vi "XMLRelult_Save_To_File2.vi"(10 "INT DATA":string[][](array[string]), 11 "XML File Path":path caption="XML文件路径") -> (2 "连接的字符串":string, 3 "XML File Path(duplicate)":path caption="XML文件路径（副本）")   [LabVIEW 2018]
uses:
  Subvi/Global.vi
panel:
  out "XML String":string caption="XML字符串"
  in  "INT DATA 3":string[][](array[string])
  in  "INT DATA 2":string[][](array[string])
  out "字符串":string
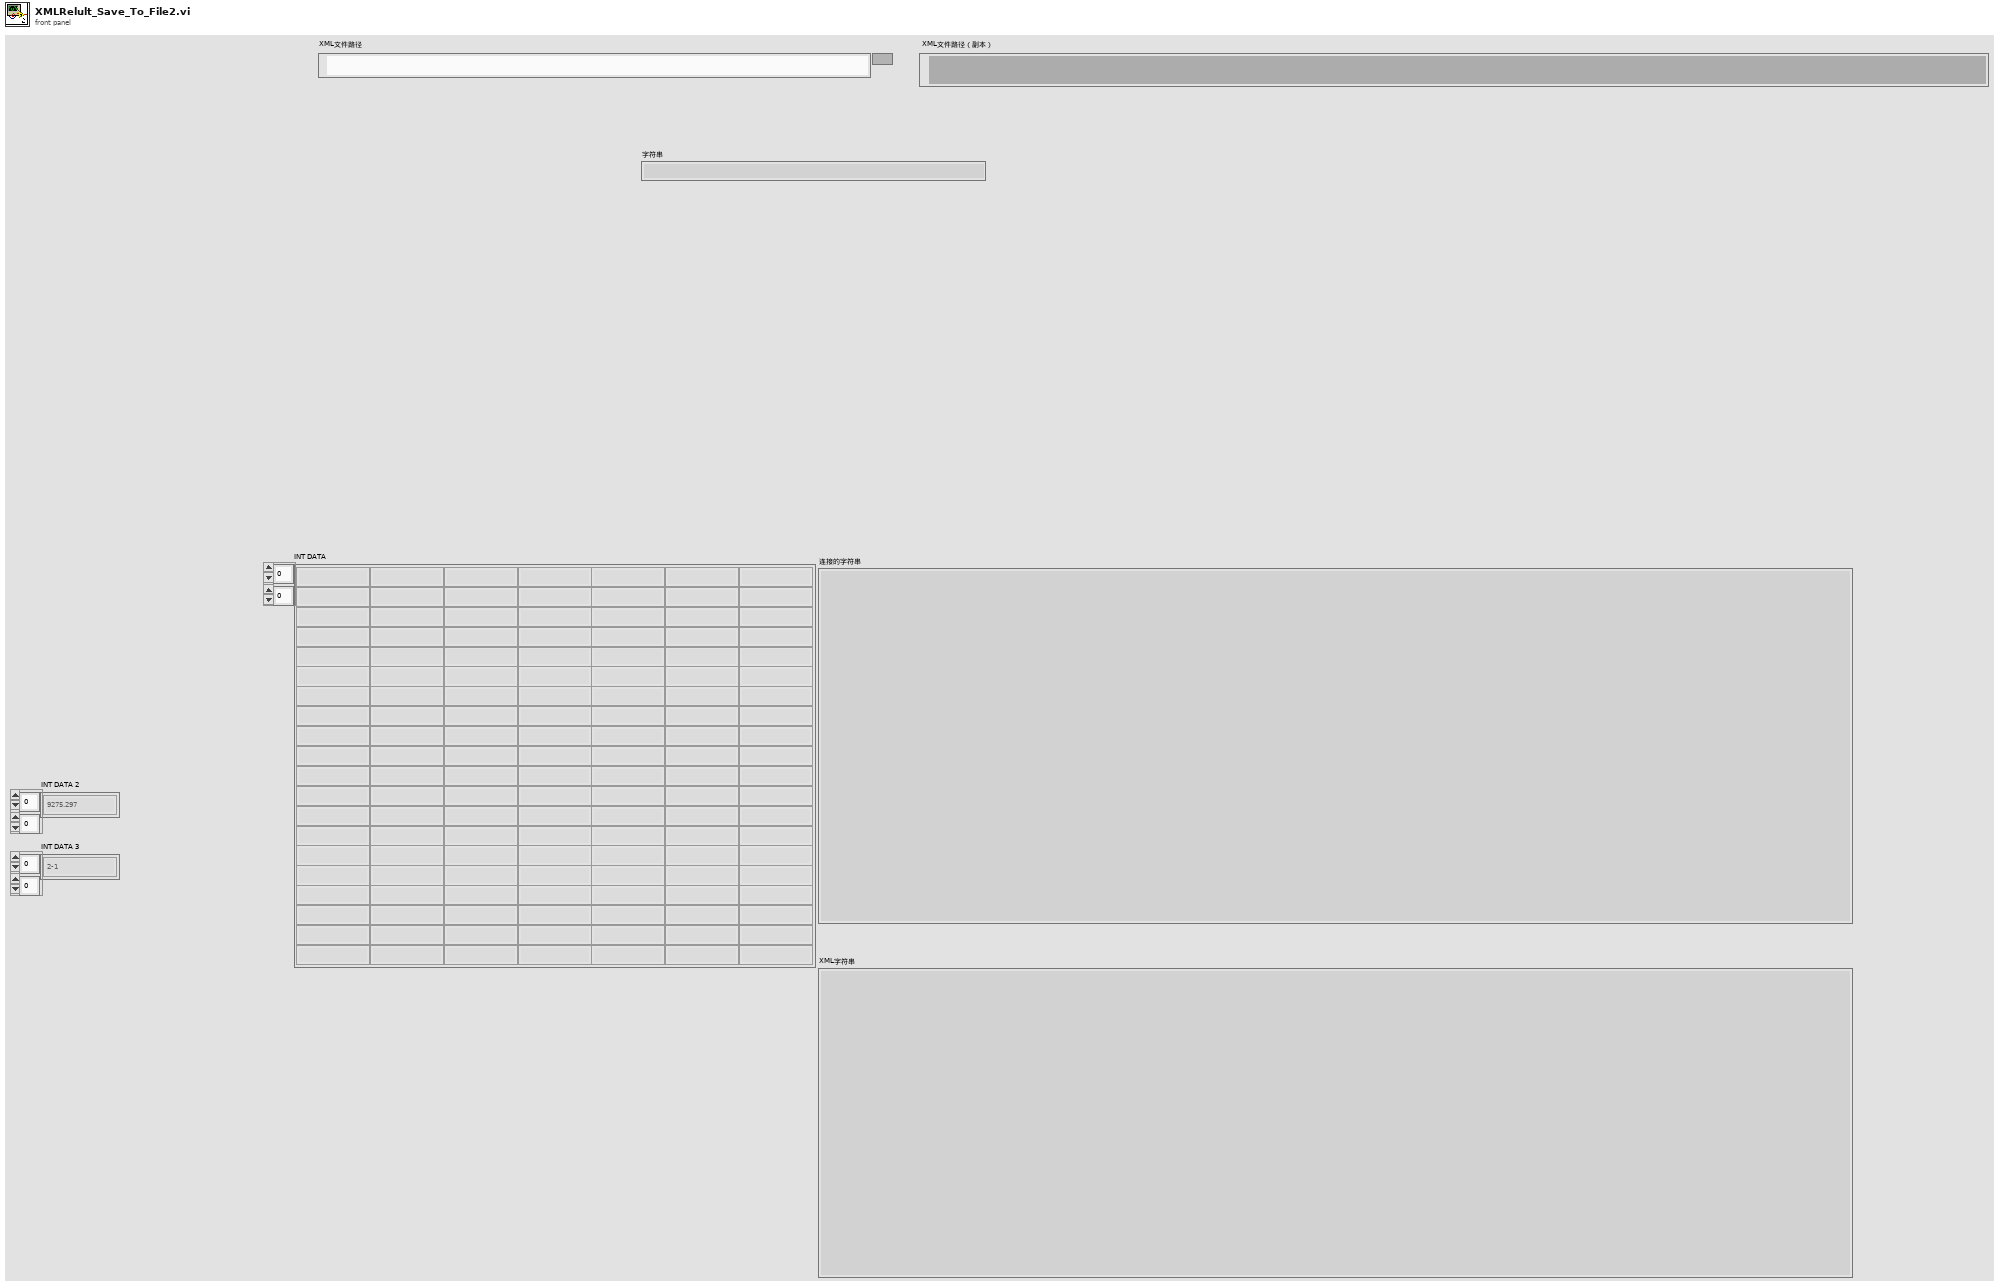
[diagram p1: front panel]
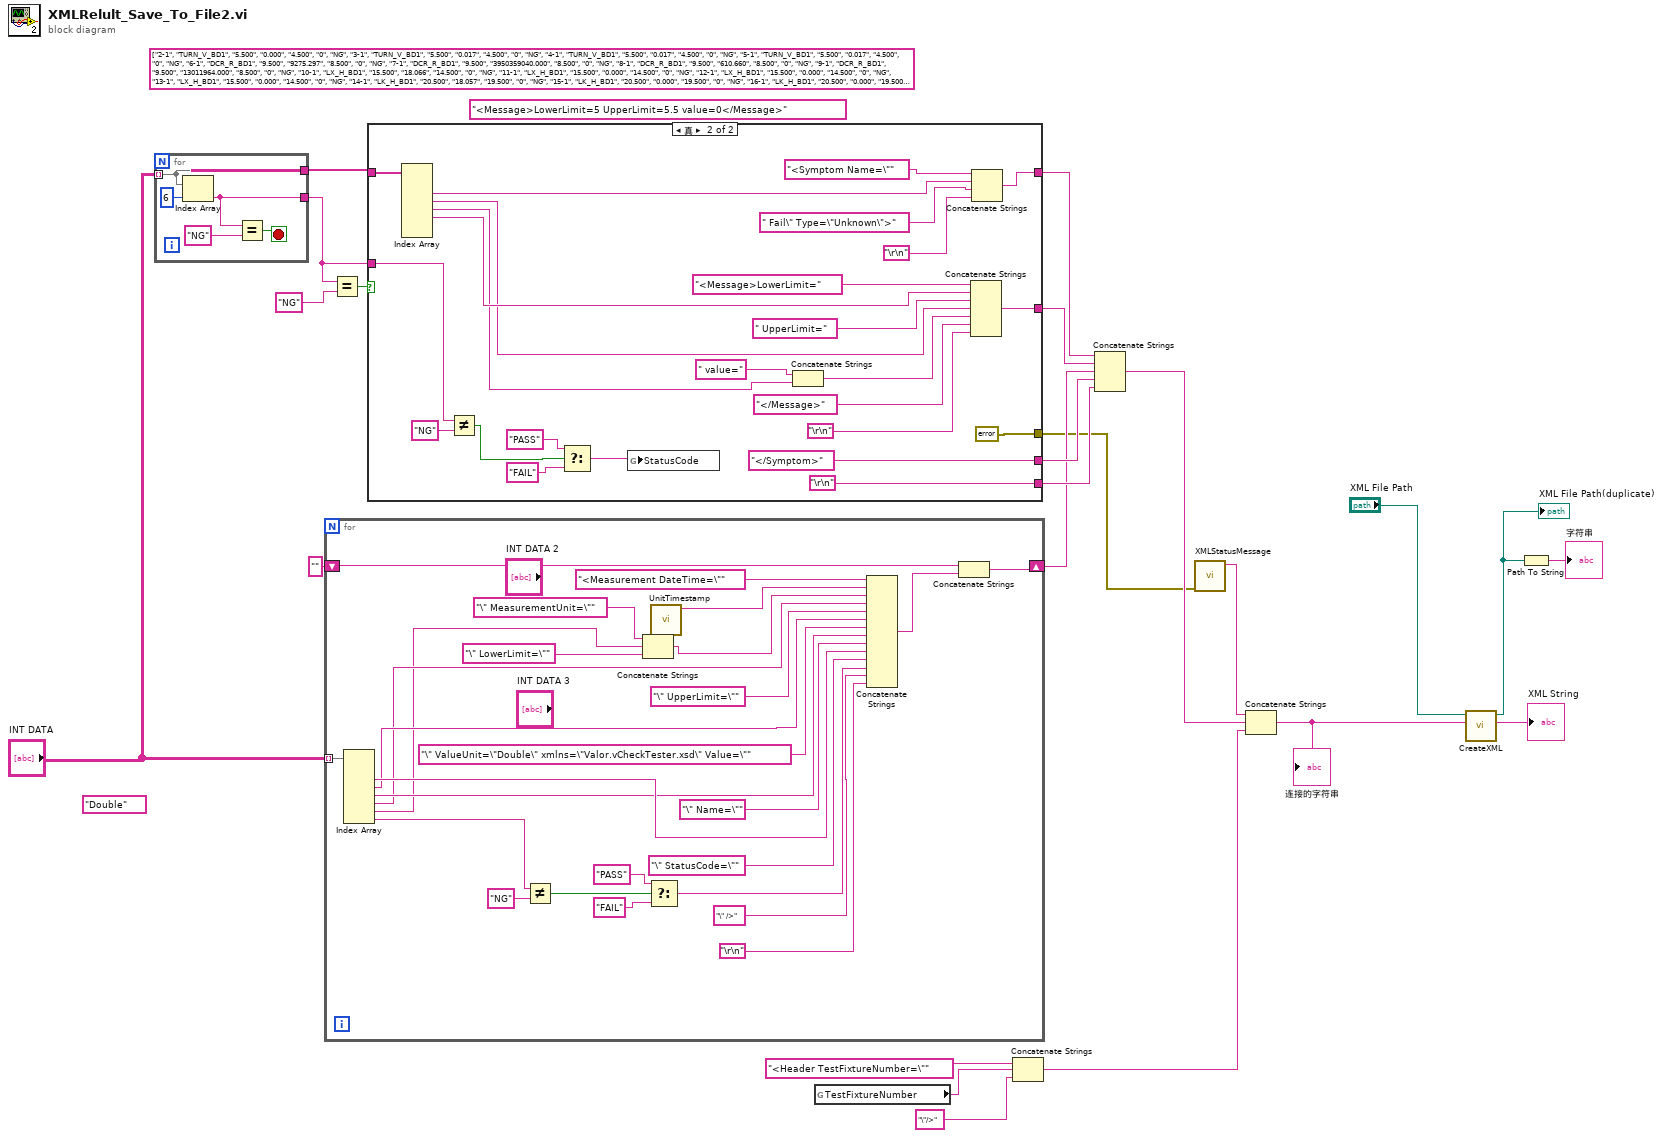
[diagram p0: block diagram]
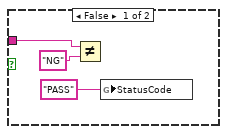
[diagram p2: hidden frame]
diagram:
  (unwired) string[][] [["2-1", "TURN_V_BD1", "5.500", "0.000", "4.500", "0", "NG"], ["3-1", "TURN_V_BD1", "5.500", "0.017", "4.500", "0", "NG"], ["4-1", "TURN_V_BD1", "5.500", "0.017", "4.500", "0", "NG"], ["5-1", "TURN_V_BD1", "5.500", "0.017", "4.500", "0", "NG"], ["6-1", "DCR_R_BD1", "9.500", "9275.297", "8.500", "0", "NG"], ["7-1", "DCR_R_BD1", "9.500", "3950359040.000", "8.500", "0", "NG"], ["8-1", "DCR_R_BD1", "9.500", "610.660", "8.500", "0", "NG"], ["9-1", "DCR_R_BD1", "9.500", "13011964.000", "8.500", "0", "NG"], ["10-1", "LX_H_BD1", "15.500", "18.066", "14.500", "0", "NG"], ["11-1", "LX_H_BD1", "15.500", "0.000", "14.500", "0", "NG"], ["12-1", "LX_H_BD1", "15.500", "0.000", "14.500", "0", "NG"], ["13-1", "LX_H_BD1", "15.500", "0.000", "14.500", "0", "NG"], ["14-1", "LK_H_BD1", "20.500", "18.057", "19.500", "0", "NG"], ["15-1", "LK_H_BD1", "20.500", "0.000", "19.500", "0", "NG"], ["16-1", "LK_H_BD1", "20.500", "0.000", "19.500", "0", "NG"], ["17-1", "LK_H_BD1", "20.500", "0.000", "19.500", "0", "NG"]] ("INT DATA")
  (unwired) "<Message>LowerLimit=5 UpperLimit=5.5 value=0</Message>"
  (unwired) "Double" ("组合框")
  n1 = for {
    tunnel: "INT DATA" -> [w25] mode=indexing
    tunnel: [w25] -> w8
    tunnel: [w24] -> w6
    stop <- w27 stop-if-true
    n2 = Index Array(array=w25, index=6 ("索引")) -> (element=w24:string)
    n3 = Equal?(x=w24, y="NG") -> (x = y?=w27:bool)
  }
  n4 = for {
    tunnel: "INT DATA" -> [w54] mode=indexing
    shift-right: [w40] -> w9
    shift-left: "" ("字符串") -> [w41]
    n5 = Index Array(array=w54) -> (element #2=w33:string, element #3=w31:string, element #4=w32:string, element #5=w30:string, element #6=w29:string, element #7=w35:string)  [unwired: 7 in, 1 out]
    n6 = Not Equal?(x=w35, y="NG") -> (x != y?=w34:bool)
    n7 = Concatenate Strings("\" MeasurementUnit=\"", w29, "\" LowerLimit=\"") -> (w53:string)
    n8 = Select(t="PASS", s=w34, f="FAIL") -> (s? t:f=w37:string)
    n9 = call "UnitTimestamp.vi"() -> ("字符串"=w43:string)  [unwired: 10 in, 1 out]
    n10 = Concatenate Strings("<Measurement DateTime=\"", w43, w53, w30, "\" UpperLimit=\"", w31, "\" ValueUnit=\"Double\" xmlns=\"Valor.vCheckTester.xsd\" Value=\"", w32, "\" Name=\"", w33, "\" StatusCode=\"", w37, "\" />", "\r\n") -> (w50:string)
    n11 = Concatenate Strings(w41, w50) -> (w40:string)
  }
  n12 = Equal?(x=w6, y="NG") -> (x = y?=w7:bool)
  n13 = case shown="真" w7 {
    tunnel: [_ w75] -> w11
    tunnel: [_ w74] -> w12
    tunnel: [_ "</Symptom>"] -> w13
    tunnel: [_ "\r\n"] -> w14
    tunnel: w8 -> [_ w71]
    tunnel: w6 -> [w56 w60]
    tunnel: [_ errorcluster {"status"=FALSE, "code"=0, "source"=""} ("error out")] -> w5
    frame False {
      n14 = Not Equal?(x=w56, y="NG") -> ()  [unwired: 1 out]
      n15 = global write "Global.vi" "StatusCode"("PASS") -> ()
    }
    frame True {
      n16 = Index Array(array=w71) -> (element #2=w70:string, element #3=w68:string, element #4=w66:string, element #5=w69:string)  [unwired: 7 in, 3 out]
      n17 = Not Equal?(x=w60, y="NG") -> (x != y?=w59:bool)
      n18 = Select(t="PASS", s=w59, f="FAIL") -> (s? t:f=w63:string)
      n19 = global write "Global.vi" "StatusCode"(w63) -> ()
      n20 = Concatenate Strings(" value=", w66) -> (w65:string)
      n21 = Concatenate Strings("<Message>LowerLimit=", w69, " UpperLimit=", w68, w65, "</Message>", "\r\n") -> (w75:string)
      n22 = Concatenate Strings("<Symptom Name=\"", w70, " Fail\" Type=\"Unknown\">", "\r\n") -> (w74:string)
    }
  }
  n23 = global read "Global.vi" "TestFixtureNumber"() -> (w21:string)
  n24 = Concatenate Strings("<Header TestFixtureNumber=\"", w21, "\"/>") -> (w18:string)
  n25 = Concatenate Strings(w12, w11, w9, w13, w14) -> (w10:string)
  n26 = call "XMLStatusMessage.vi"("error in (no error)"=w5) -> ("连接的字符串"=w19:string)  [unwired: 9 in, 1 out]
  n27 = Concatenate Strings(w19, w10, w18) -> (w20:string)
  "连接的字符串" <- w20
  n28 = call "CreateXML.vi"("XML Input"=w20, "XML File Path"="XML File Path") -> ("XML String"=→"XML String":string, "XML File Path(duplicate)"=w3:path)  [unwired: 7 in, 1 out]
  "XML File Path(duplicate)" <- w3
  n29 = Path To String(path=w3) -> (string=→"字符串":string)
